vi "AdjustAll (Chris Bonomi's conflicted copy 2015-03-17).vi"(0 "SteeringAngleArray":dbl[](array[numeric]), 2 "PowerArray":dbl[](array[numeric]), 8 "Third Speed":bool, 9 "JoystickValues":dbl[](array[numeric]), 10 "FL Enc":dbl, 11 "EncoderTicksPerRev":dbl=1988.0, 12 "FR Enc":dbl, 14 "BL Enc":dbl, 15 "Gain":dbl=50.0, 16 "BR Enc":dbl, 17 "Shaping Degree":dbl=2.0, 18 "20% Speed":bool) -> (20 "FL Set Out":dbl, 21 "FR Set Out":dbl, 22 "BL Set Out":dbl, 23 "BR Set Out":dbl, 24 "FL Power":dbl, 25 "FR Power":dbl, 26 "BL Power":dbl, 27 "BR Power":dbl)   [LabVIEW 2014]
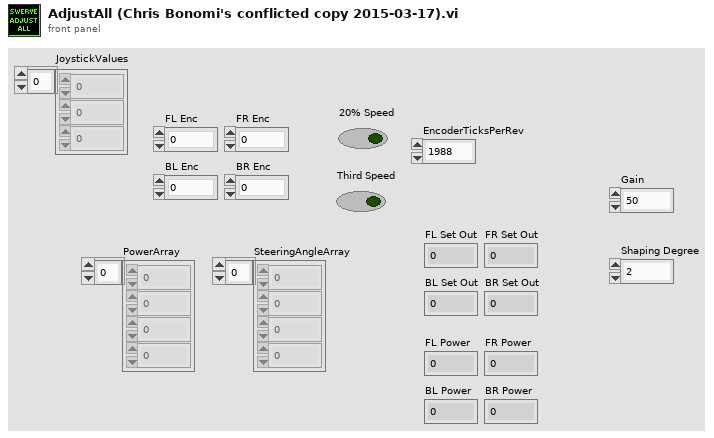
[diagram p1: front panel]
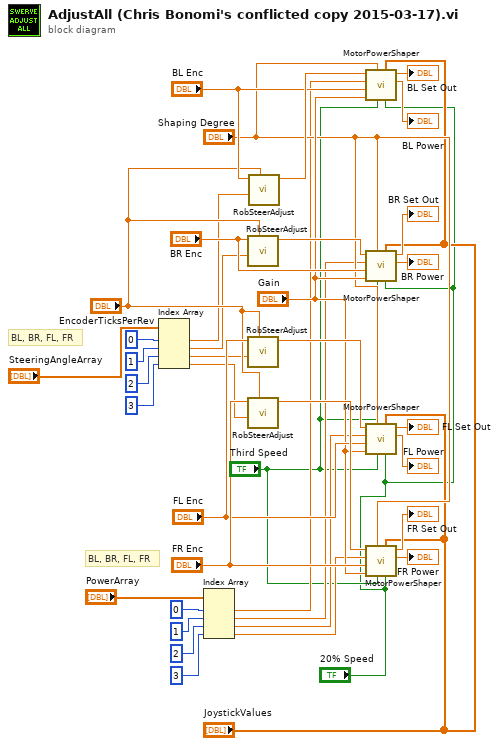
[diagram p0: block diagram]
diagram:
  # "BL, BR, FL, FR"
  # "BL, BR, FL, FR"
  n1 = Index Array(array="SteeringAngleArray", index #1=0 ("index"), index #2=1 ("index"), index #3=2 ("index"), index #4=3 ("index")) -> (element #1=w15:dbl, element #2=w14:dbl, element #3=w13:dbl, element #4=w12:dbl)
  n2 = Index Array(array="PowerArray", index #1=0 ("index"), index #2=1 ("index"), index #3=2 ("index"), index #4=3 ("index")) -> (element #1=w6:dbl, element #2=w5:dbl, element #3=w4:dbl, element #4=w3:dbl)
  n3 = call "RobSteerAdjust.vi"("EncoderTicksPerRev"="EncoderTicksPerRev", "Set In"=w14, "Encoder"="BR Enc") -> ("Set Out"=w38:dbl)  [unwired: 8 in]
  n4 = call "RobSteerAdjust.vi"("EncoderTicksPerRev"="EncoderTicksPerRev", "Set In"=w13, "Encoder"="FL Enc") -> ("Set Out"=w34:dbl)  [unwired: 8 in]
  n5 = call "RobSteerAdjust.vi"("EncoderTicksPerRev"="EncoderTicksPerRev", "Set In"=w12, "Encoder"="FR Enc") -> ("Set Out"=w40:dbl)  [unwired: 8 in]
  n6 = call "RobSteerAdjust.vi"("EncoderTicksPerRev"="EncoderTicksPerRev", "Set In"=w15, "Encoder"="BL Enc") -> ("Set Out"=w36:dbl)  [unwired: 8 in]
  n7 = call "MotorPowerShaper.vi"("20% Speed"="20% Speed", "JoystickValues"="JoystickValues", "Third Speed"="Third Speed", "Shaping Degree"="Shaping Degree", "Gain"="Gain", "Position"="BL Enc", "Power"=w6, "Setpoint"=w36) -> ("Power Out"=→"BL Power":dbl, "Setpoint Out"=→"BL Set Out":dbl)  [unwired: 2 in]
  n8 = call "MotorPowerShaper.vi"("20% Speed"="20% Speed", "JoystickValues"="JoystickValues", "Third Speed"="Third Speed", "Shaping Degree"="Shaping Degree", "Gain"="Gain", "Position"="BR Enc", "Power"=w5, "Setpoint"=w38) -> ("Power Out"=→"BR Power":dbl, "Setpoint Out"=→"BR Set Out":dbl)  [unwired: 2 in]
  n9 = call "MotorPowerShaper.vi"("20% Speed"="20% Speed", "JoystickValues"="JoystickValues", "Third Speed"="Third Speed", "Shaping Degree"="Shaping Degree", "Gain"="Gain", "Position"="FL Enc", "Power"=w4, "Setpoint"=w34) -> ("Power Out"=→"FL Power":dbl, "Setpoint Out"=→"FL Set Out":dbl)  [unwired: 2 in]
  n10 = call "MotorPowerShaper.vi"("20% Speed"="20% Speed", "JoystickValues"="JoystickValues", "Third Speed"="Third Speed", "Shaping Degree"="Shaping Degree", "Gain"="Gain", "Position"="FR Enc", "Power"=w3, "Setpoint"=w40) -> ("Power Out"=→"FR Power":dbl, "Setpoint Out"=→"FR Set Out":dbl)  [unwired: 2 in]
